vi "Decorator.vi"(10 "jettl":refnum<class "jettl.lvclass">, 11 "Base jettl in":refnum<class "Base jettl.lvclass">) -> (3 "Base jettl out":refnum<class "Base jettl.lvclass">)   [LabVIEW 2021, in "jettl.lvlib" / "Base jettl.lvclass"]
uses:
  Base jettl.lvclass
  jettl/jettl.lvclass
  Base jettl.lvclass/Base jettl.ctl
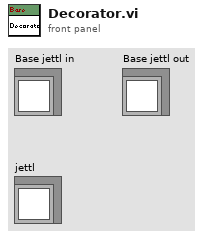
[diagram p1: front panel]
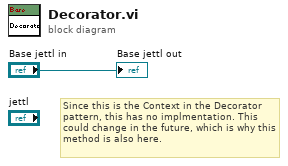
[diagram p0: block diagram]
diagram:
  # "Since this is the Context in the Decorator pattern, this has no implmentation. This could change in the future, which is why this method is also here."
  "Base jettl out" <- "Base jettl in"
